vi "AMWave.vi"(10 "Waveform Parameters":T1, 11 "Digitizing Parameters":T2) -> (3 "Graph Outputs":cluster{"Time":dbl[], "Displacement":dbl[]})   [LabVIEW 2014]
uses:
  <vilib>/imath/engines/lvmath2/RunTimeEngine/Managers/WorkSpace/UID Generator.vi
  <vilib>/imath/engines/lvmath2/RunTimeEngine/RunTimeType/NIMS_RunTimeType_From StrictType (excl LVString).vi
  <instcachedir>/0/NIMS_RunTimeType_From StrictType (excl LVString)_6F30FCEAD152B34FB6BC3D48AAFE00E6.lvgen/NIMS_RunTimeType_From StrictType (excl LVString)_6F30FCEAD152B34FB6BC3D48AAFE00E6_000.vi
  <vilib>/imath/engines/lvmath2/RunTimeEngine/LocalVariableDefStatement/MC_LocalVariableDefStatement_Display.vi
  <vilib>/imath/engines/lvmath2/RunTimeEngine/RangeToken/NIMS_Range.vi
  <instcachedir>/0/NIMS_Range_6DDDFF7386AB584A9063FA25EAF603C1.lvgen/NIMS_Range_6DDDFF7386AB584A9063FA25EAF603C1_000.vi
  <vilib>/imathl/engines/lvmath/Functions/Error Handling/Create Error.vi
  <vilib>/imath/engines/lvmath2/RunTimeEngine/ArithmeticOperatorToken/NIMS_ArithmeticOperator_times.vi
  <instcachedir>/0/NIMS_ArithmeticOperator_times_831F30C6BFCCF94698B6F46369084E97.lvgen/NIMS_ArithmeticOperator_times_831F30C6BFCCF94698B6F46369084E97_000.vi
  <vilib>/imath/engines/lvmath2/RunTimeEngine/Managers/SymbolTable/Clear UID.vi
  <vilib>/imath/engines/lvmath2/RunTimeEngine/NodeEndStatement/NIMS_NodeEndStatement_Output.vi
  <instcachedir>/0/NIMS_NodeEndStatement_Output_53EC0D466D134D7ABD903AC30B43404B.lvgen/NIMS_NodeEndStatement_Output_53EC0D466D134D7ABD903AC30B43404B_005.vi
  <vilib>/imath/engines/lvmath2/RunTimeEngine/ErrorHandling/NIMS_Finalize Error.vi
  <vilib>/imath/engines/lvmath2/RunTimeEngine/Managers/SymbolTable/NIMS_WorkSpace.lvlib
panel:
  out "XY Graph":cluster{"t":dbl[], "x":dbl[]}(graph)
  # "Parameters controlling\nwaveform  signal\nsampling"
  # "X and Y var. indicators"
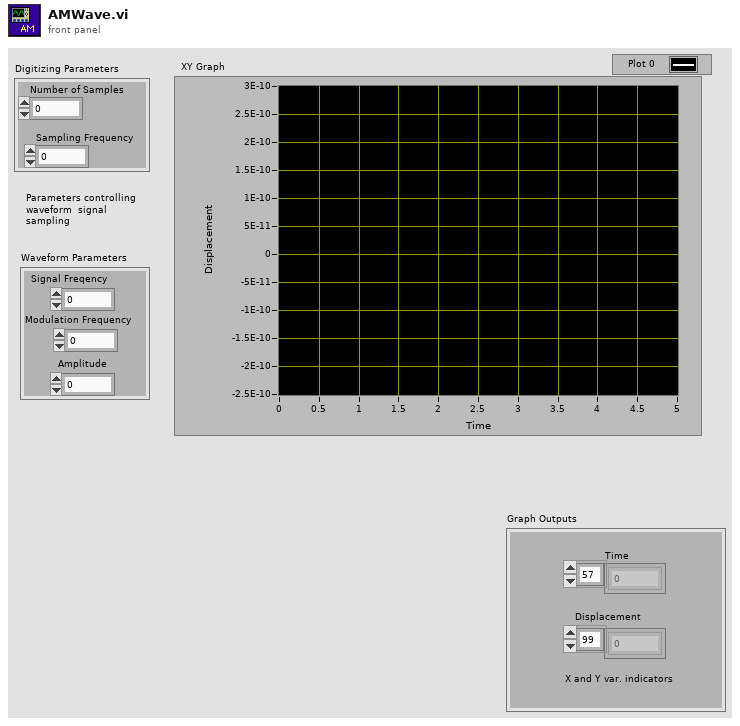
[diagram p1: front panel]
types:
  T1 = cluster{"Signal Freqency":dbl, "Modulation Frequency":dbl, "Amplitude":dbl}
  T2 = cluster{"Number of Samples":dbl, "Sampling Frequency":dbl}
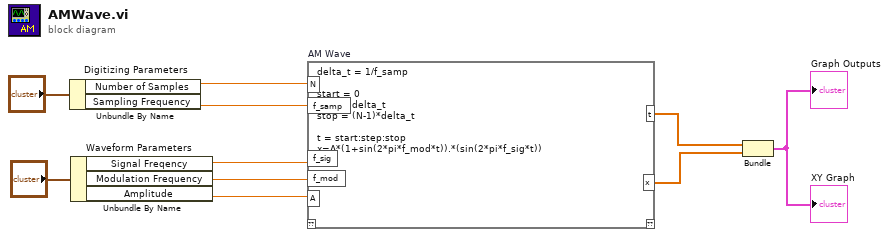
[diagram p0: block diagram]
diagram:
  n1 = Unbundle By Name("Digitizing Parameters") -> ("Number of Samples"=w9:dbl, "Sampling Frequency"=w8:dbl)
  n2 = Unbundle By Name("Waveform Parameters") -> ("Signal Freqency"=w6:dbl, "Modulation Frequency"=w5:dbl, "Amplitude"=w4:dbl)
  n3 = mathscript code="delta_t = 1/f_samp\n\nstart = 0\nstep = delta_t\nstop = (N-1)*delta_t\n\nt = start:step:stop\nx=A*(1+sin(2*pi*f_mod*t)).*(sin(2*pi*f_sig*t))" "AM Wave"("f_samp"=w8, "f_sig"=w6, "A"=w4, "N"=w9, "f_mod"=w5) -> ("x"=w3:dbl[], "t"=w2:dbl[])  [unwired: 1 in, 1 out]
  n4 = Bundle("t"=w2, "x"=w3) -> (→"XY Graph" →"Graph Outputs":cluster{"t":dbl[], "x":dbl[]})  [unwired: 1 in]
